vi "RSZVB Set IMOD Measurement Order.vi"(7 "Measurement State (T: On)":bool=TRUE, 8 "error in (no error)":errorcluster {"code" format="%.0x"}, 9 "Product Order (3)":i32(ring)=3 items=["3"=3, "5"=5, "7"=7, "9"=9], 10 "Channel (1)":i32=1, 11 "VISA session":refnum<visa-resource-name>) -> (0 "error out":errorcluster {"code" format="%.0x"}, 3 "dup VISA session":refnum<visa-resource-name>)   [LabVIEW 2011]
doc: "This VI enables or disables the measurement of the intermodulation products of order <IM order>.\n\nNote(s):\n\n(1) This VI is not available for R&S ZVB instrument.\n\nRemote-control command(s):\n[SENSe<Ch>:]FREQuency:IMODulation:ORDer<Im>[:STATe] ON | OFF"
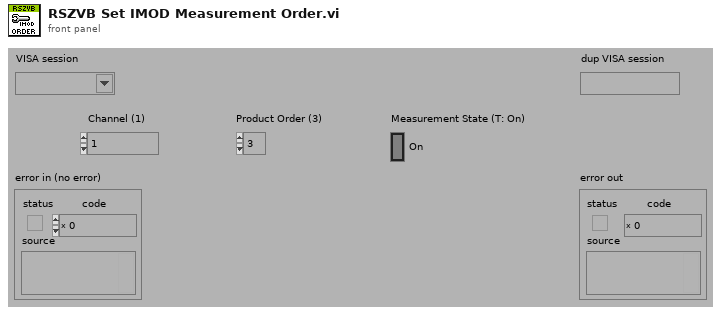
[diagram p1: front panel]
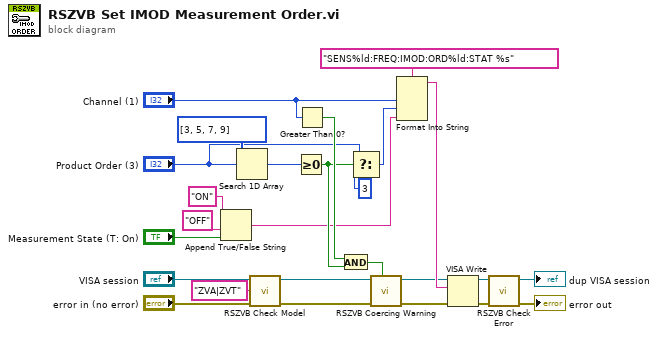
[diagram p0: block diagram]
diagram:
  n1 = Append True/False String(1:"Measurement State (T: On)", 2:"OFF" ("false string"), 3:"ON" ("true string")) -> (0:w10:string)  [unwired: 1 in]
  n2 = Search 1D Array(1D array=i32[] [3, 5, 7, 9], element="Product Order (3)") -> (index of element=w7:i32)  [unwired: 1 in]
  n3 = call "RSZVB Check Model.vi"("error in (no error)"="error in (no error)", "Model"="ZVA|ZVT", "VISA session"="VISA session") -> ("error out"=w4:errorcluster, "dup VISA session"=w5:refnum<visa-resource-name>)  [unwired: 7 in]
  n4 = Greater Or Equal To 0?(x=w7) -> (x >= 0?=w16:bool)
  n5 = Greater Than 0?(x="Channel (1)") -> (x > 0?=w18:bool)
  n6 = And(x=w18, y=w16) -> (x .and. y?=w17:bool)
  n7 = Select(t="Product Order (3)", s=w16, f=3) -> (s? t:f=w14:i32)
  n8 = call "RSZVB Coercing Warning.vi"("In Range?"=w17, "error in (no error)"=w4, "VISA session"=w5) -> ("error out"=w23:errorcluster, "dup VISA session"=w22:refnum<visa-resource-name>)  [unwired: 7 in]
  n9 = Format Into String(format string="SENS%ld:FREQ:IMOD:ORD%ld:STAT %s", "Channel (1)", w14, w10) -> (resulting string=w24:string)  [unwired: 2 in, 1 out]
  n10 = VISA Write(VISA resource name=w22, write buffer=w24, error in (no error)=w23) -> (VISA resource name out=w25:refnum<visa-resource-name>, error out=w26:errorcluster)  [unwired: 1 out]
  n11 = call "RSZVB Check Error.vi"("error in (no error)"=w26, "VISA session"=w25) -> ("error out"=→"error out":errorcluster, "dup VISA session"=→"dup VISA session":refnum<visa-resource-name>)  [unwired: 8 in]
